vi "TWM Client Cmd Get Status.vi"(5 "timeout [ms] (3000)":i32=3000, 7 "end of packet key":string="TWM:command:EndOfPacket", 8 "error in":errorcluster, 10 "clear errors? (False)":bool, 11 "handle":i32) -> (0 "error out":errorcluster, 1 "error message":string, 2 "ready?":bool, 3 "handle out":i32, 4 "status string":string)   [LabVIEW 2020, in "TWM Client.lvlib"]
doc: "Write Get status command packet to TWM server. Get answer. Returns 'Ready?', when server is ready to do stuff. Also returns optional error text message from server. It will generate error if error message was not empty."
uses:
  TWM Client.lvlib
  octave/infolib/GetString.vi
  octave/infolib/Get 1D String.vi
  <vilib>/Utility/error.llb/Error Cluster From Error Code.vi
  octave/infolib/Boolean.vi
  <vilib>/ErrorRing/Error Ring.xnode
  octave/infolib/infolib.lvlib
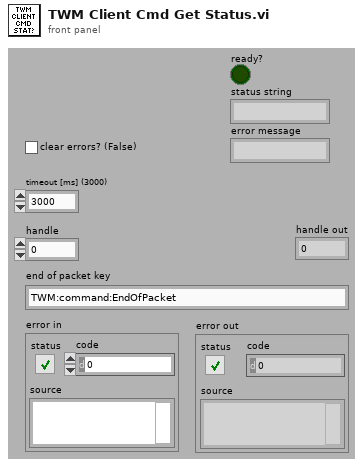
[diagram p1: front panel]
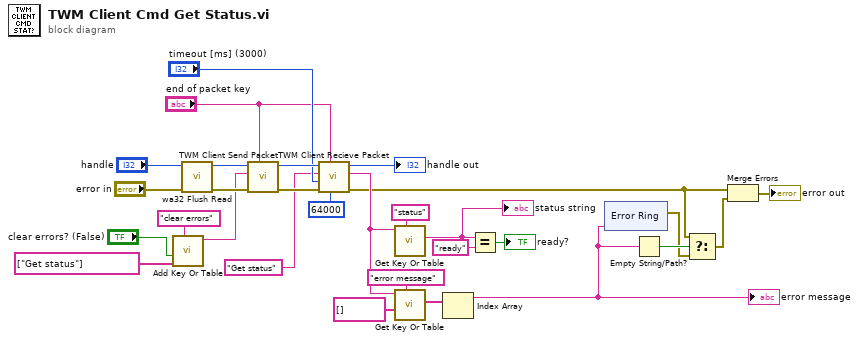
[diagram p0: block diagram]
diagram:
  n1 = call-poly "Add Key Or Table.vi"("key description"="clear errors", "sections"=string[] ["Get status"], "boolean"="clear errors? (False)") -> ("info data out"=w1:string)  [unwired: 7 in, 1 out]
  n2 = call "wa32 Flush Read.vi"("error in"="error in", "handle"="handle") -> ("error out"=w7:errorcluster, "handle out"=w6:i32)  [unwired: 7 in, 1 out]
  n3 = call "TWM Client Send Packet.vi"("end of packet key"="end of packet key", "error in"=w7, "command string"=w1, "handle"=w6) -> ("error out"=w23:errorcluster, "handle out"=w21:i32)  [unwired: 6 in]
  n4 = call "TWM Client Recieve Packet.vi"("max message length (1024)"=64000, "end of packet key"="end of packet key", "error in"=w23, "timeout [ms] (5000 ms)"="timeout [ms] (3000)", "message header (empty)"="Get status" ("key string"), "handle in"=w21) -> ("error out"=w11:errorcluster, "message data"=w16:string, "handle out"=→"handle out":i32)  [unwired: 3 in]
  n5 = call-poly "Get Key Or Table.vi"("key description"="status", "info data"=w16) -> ("value"=w28:string)  [unwired: 6 in, 3 out]
  "status string" <- w28
  n6 = call-poly "Get Key Or Table.vi"("key description"="error message", "string"=string[] [], "info data"=w16) -> ("value"=w24:string[])  [unwired: 5 in, 3 out]
  n7 = Index Array(array=w24) -> (element=w13:string)  [unwired: 1 in]
  "error message" <- w13
  n8 = Equal?(x=w28, y="ready") -> (x = y?=→"ready?":bool)
  n9 = xnode "Error Ring"("parameter 0"=w13) -> ("error out"=w12:errorcluster)
  n10 = Empty String/Path?(string/path=w13) -> (empty?=w14:bool)
  n11 = Select(t=w11, s=w14, f=w12) -> (s? t:f=w10:errorcluster)
  n12 = Merge Errors(w11, w10) -> (→"error out":errorcluster)
